vi "GEOM_Read_ReadModes.vi"(8 "error in (no error)":errorcluster, 10 "Detector Format":string, 11 "file path":path) -> (0 "error out":errorcluster, 2 "ReadModes":T1[](array[typedef]) {"amplifiers"."fliped" items=["none", "horizontal", "vertical"]; "amplifiers"."type" items=["LL", "LR", "UL", "UR"]}, 3 "file path out":path, 4 "ydata":i32, 6 "xdata":i32)   [LabVIEW 2016]
uses:
  GEOM_ReadMode.ctl
  GEOM_Amplifier.ctl
  GEOM_AmpType.ctl
  GEOM_ROI.ctl
  GEOM_Coords.ctl
  <vilib>/Utility/config.llb/Read Key (String).vi
  <vilib>/Utility/config.llb/NI_LVConfig.lvlib
panel:
  in  "ReadMode":T1 {"amplifiers"."fliped" items=["none", "horizontal", "vertical"]; "amplifiers"."type" items=["LL", "LR", "UL", "UR"]}
  in  "section":string="READMODES"
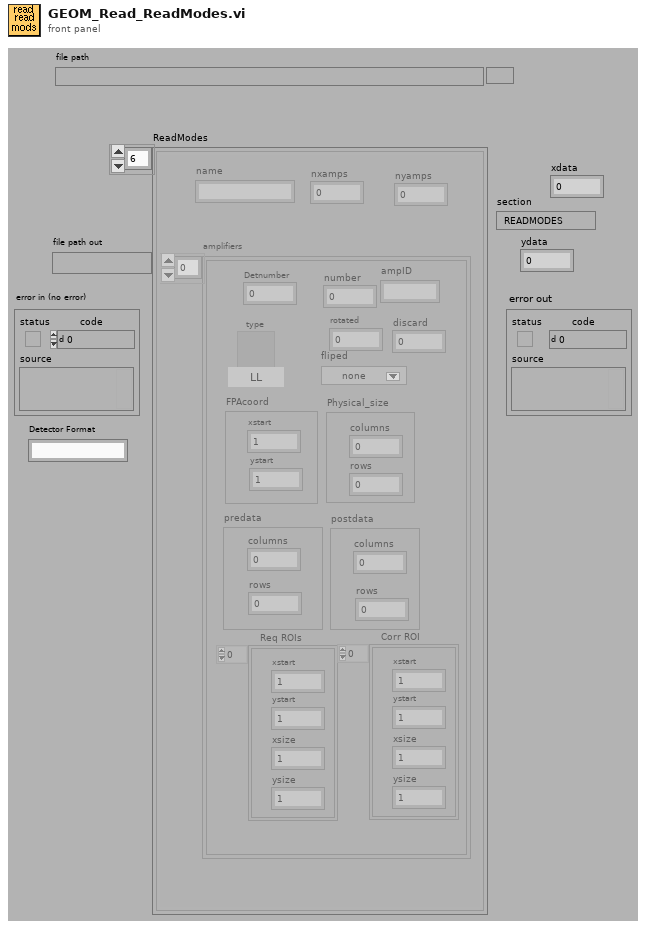
[diagram p1: front panel]
types:
  T1 = typedef "GEOM_ReadMode.ctl" = cluster{"name":string, "amplifiers":T2[], "nxamps":i32, "nyamps":i32}
  T2 = typedef "GEOM_Amplifier.ctl" = cluster{"number":i32, "type":T3, "rotated":i16, "fliped":u16, "FPAcoord":cluster{"xstart":i32, "ystart":i32}, "Physical_size":cluster{"columns":i32, "rows":i32}, "predata":cluster{"columns":i32, "rows":i32}, "postdata":cluster{"columns":i32, "rows":i32}, "Req ROIs":T4, "Corr ROI":T4, "Detnumber":i32, "ampID":string, "discard":i32}
  T3 = typedef "GEOM_AmpType.ctl" = u16
  T4 = typedef "GEOM_ROI.ctl" = T5[]
  T5 = typedef "GEOM_Coords.ctl" = cluster{"xstart":u32, "ystart":u32, "xsize":u32, "ysize":u32}
  T6 = typedef "NI_LVConfig.lvlib/Config Data RefNum.ctl" = refnum<k1>
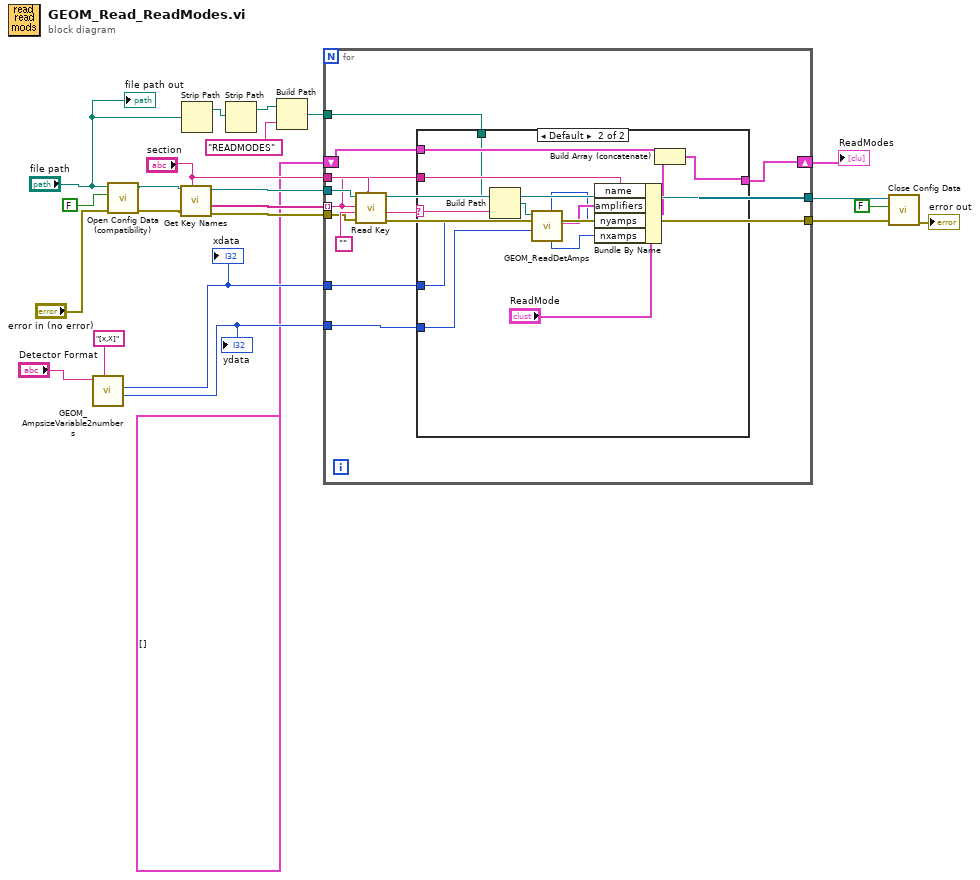
[diagram p0: block diagram]
diagram:
  n1 = call "GEOM_AmpsizeVariable2numbers.vi"("separator"="[x,X]", "ampval"="Detector Format") -> ("amprows"=w8:i32, "ampcols"=w9:i32)  [unwired: 2 in, 6 out]
  "xdata" <- w9
  "ydata" <- w8
  n2 = call <vilib>:"Open Config Data (compatibility).vi"("error in (no error)"="error in (no error)", "create file if necessary (T)"=FALSE ("create file if necessary? (T)"), "configuration file path"="file path") -> ("error out"=w21:errorcluster, "refnum"=w22:T6)  [unwired: 6 in, 1 out]
  n3 = call <vilib>:"Get Key Names.vi"("section"="section", "error in (no error)"=w21, "refnum"=w22) -> ("error out"=w17:errorcluster, "key names"=w20:string[], "refnum out"=w19:T6)  [unwired: 6 out]
  n4 = Strip Path(path="file path") -> (stripped path=w6:path)  [unwired: 1 out]
  n5 = Strip Path(path=w6) -> (stripped path=w5:path)  [unwired: 1 out]
  n6 = Build Path(base path=w5, name or relative path="READMODES" ("string")) -> (appended path=w3:path)
  n7 = for {
    tunnel: w20 -> [w33] mode=indexing
    tunnel: "section" -> [w36]
    tunnel: w19 -> [w35]
    shift-right: [w27] -> w2
    shift-left: T1[] [] -> [w32]
    tunnel: [w31] -> w18
    tunnel: w17 -> [w30]
    tunnel: [w29] -> w16
    tunnel: w9 -> [w26]
    tunnel: w8 -> [w25]
    tunnel: w3 -> [w24]
    n8 = call-poly <vilib>:"Read Key.vi"("section"=w36, "error in (no error)"=w30, "default value"="", "key"=w33, "refnum"=w35) -> ("error out"=w29:errorcluster, "value"=w28:string, "refnum out"=w31:T6)  [unwired: 1 in, 3 out]
    n9 = case shown="Default" w28 {
      selector: w28 -> [_ w42]
      tunnel: w33 -> [_ w44]
      tunnel: w32 -> [w37 w47]
      tunnel: [w37 w48] -> w27
      tunnel: w26 -> [_ w46]
      tunnel: w25 -> [_ w45]
      tunnel: w24 -> [_ w43]
      frame "", " " {
      }
      frame Default {
        n10 = Build Path(base path=w43, name or relative path=w42) -> (appended path=w41:path)
        n11 = call "GEOM_ReadDetAmps.vi"("detrows"=w45, "detcols"=w46, "file path"=w41) -> ("amplifiers"=w50:T2[], "numxamps"=w38:i32, "numyamps"=w39:i32)  [unwired: 1 in, 5 out]
        n12 = Bundle By Name(cluster="ReadMode", "name"=w44, "amplifiers"=w50, "nyamps"=w39, "nxamps"=w38) -> (w49:T1)
        n13 = Build Array (concatenate)(w47, w49) -> (w48:T1[])
      }
    }
  }
  "ReadModes" <- w2
  n14 = call <vilib>:"Close Config Data.vi"("error in (no error)"=w16, "write file if changed (T)"=FALSE ("write configuration file? (F)"), "refnum"=w18) -> ("error out"=→"error out":errorcluster)  [unwired: 8 out]
  "file path out" <- "file path"
